vi "NanoScan Get Number.vi"(0 "VISA Ref":refnum<visa-resource-name>, 7 "Reply":string, 11 "Error In":errorcluster) -> (4 "VISA Ref Dup":refnum<visa-resource-name>, 8 "Number":dbl, 15 "Error Out":errorcluster)   [LabVIEW 2020]
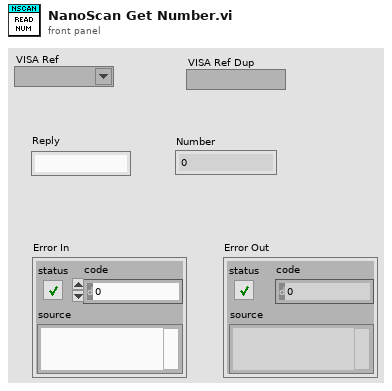
[diagram p1: front panel]
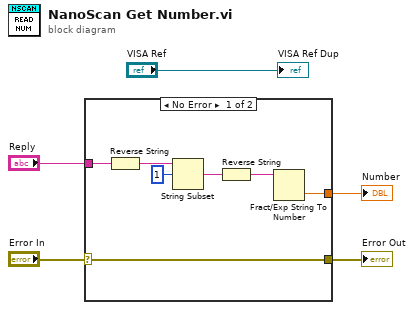
[diagram p0: block diagram]
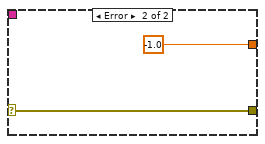
[diagram p2: hidden frame]
diagram:
  n1 = case shown="No Error" "Error In" {
    selector: "Error In" -> [w6 w14]
    tunnel: "Reply" -> [w12 _]
    tunnel: [w6 w14] -> w2
    tunnel: [w7 -1.0] -> w1
    frame No Error {
      n2 = Reverse String(1:w12) -> (0:w11:string)
      n3 = String Subset(string=w11, offset (0)=1) -> (substring=w9:string)  [unwired: 1 in]
      n4 = Reverse String(1:w9) -> (0:w8:string)
      n5 = Fract/Exp String To Number(string=w8) -> (number=w7:dbl)  [unwired: 3 in, 1 out]
    }
    frame Error {
    }
  }
  "Number" <- w1
  "Error Out" <- w2
  "VISA Ref Dup" <- "VISA Ref"
